vi "Keithley 6517 Linear Calculation.vi"() -> ()   [LabVIEW 2016]
doc: "Executes a Linear Calculation and reads the result.\n\n<B>Note:</B>\nThis Example is ONLY compatible with model 6514."
uses:
  <instrlib>/Keithley 6517/Keithley 6517.lvlib
panel:
  out "Linear Calculation Result":dbl
  in  "Offset (b) Value (0.000000)":dbl
  in  "Scale Factor (m) Value (1.000000)":dbl=1.0
  in  "VISA resource name":refnum<visa-resource-name>
  # "(c) 2016-2017 National Instruments.  ALL RIGHTS RESERVED."
  # "Note: This Example is ONLY compatible with model 6514."
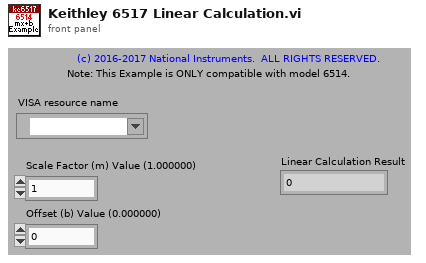
[diagram p1: front panel]
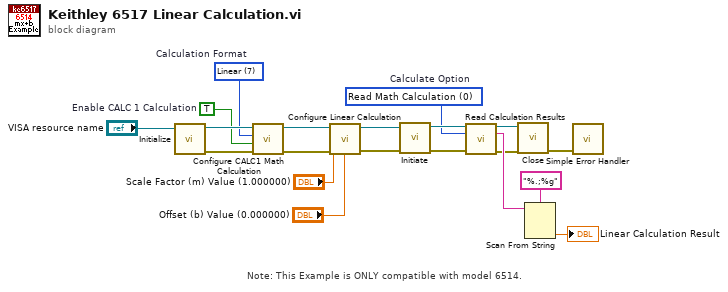
[diagram p0: block diagram]
diagram:
  w7 = 0 items=["Read Math Calculation", "Recalculate Math Calculation", "Read Buffer Data Calculation", "Read Limit Tests"]  # Calculate Option
  w16 = TRUE  # Enable CALC 1 Calculation
  w17 = 7 items=["NONE", "Percent", "Polynomial", "Ratio", "Deviation", "Percent deviation", "Logarithmic base 10", "Linear"]  # Calculation Format
  # "Note: This Example is ONLY compatible with model 6514."
  n1 = call <instrlib>:"Initialize.vi"("VISA resource name"="VISA resource name") -> ("error out"=w19:errorcluster, "VISA resource name out"=w18:refnum<visa-resource-name>)  [unwired: 9 in]
  n2 = call <instrlib>:"Configure CALC1 Math Calculation.vi"("error in (no error)"=w19, "Enable CALC 1 Calculation (T: Enable)"=w16, "Calculation Format (2: Polynomial)"=w17, "VISA resource name"=w18) -> ("error out"=w15:errorcluster, "VISA resource name out"=w14:refnum<visa-resource-name>)  [unwired: 6 in]
  n3 = call <instrlib>:"Configure Linear Calculation.vi"("error in (no error)"=w15, "Offset (b) Value (0.000000)"="Offset (b) Value (0.000000)", "Scale Factor (m) Value (1.000000)"="Scale Factor (m) Value (1.000000)", "VISA resource name"=w14) -> ("error out"=w11:errorcluster, "VISA resource name out"=w10:refnum<visa-resource-name>)  [unwired: 6 in]
  n4 = call <instrlib>:"Initiate.vi"("error in (no error)"=w11, "VISA resource name"=w10) -> ("error out"=w9:errorcluster, "VISA resource name out"=w8:refnum<visa-resource-name>)  [unwired: 8 in]
  n5 = call <instrlib>:"Read Calculation Results.vi"("VISA resource name"=w8, "Calculate Option (0: Read Math Calculation)"=w7, "error in (no error)"=w9) -> ("VISA resource name out"=w2:refnum<visa-resource-name>, "Math Calculation Result"=w6:string, "error out"=w3:errorcluster)  [unwired: 6 in, 4 out]
  n6 = call <instrlib>:"Close.vi"("error in (no error)"=w3, "VISA resource name"=w2) -> ("error out"=w1:errorcluster)  [unwired: 9 in]
  n7 = Scan From String(format string="%.;%g", input string=w6) -> (output 1=→"Linear Calculation Result":dbl)  [unwired: 3 in, 3 out]
  n8 = call <vilib>:"Simple Error Handler.vi"("error in (no error)"=w1) -> ()  [unwired: 4 in, 5 out]
